vi "VIQA Audit.vi"(6 "Abort":refnum<vi>, 7 "Ignore":T1, 8 "error in (no error)":errorcluster, 9 "AuditSlide":refnum<vi>, 10 "AuditMCLB":refnum<vi>, 11 "My Computer":refnum<vi>) -> (0 "error out":errorcluster, 3 "Audit":T2[](array[typedef]))   [LabVIEW 2018, in "VI Quality.lvlib"]
doc: "This VI audits the project items given the filter criteria"
uses:
  VI Quality.lvlib
  Controls/VIQA Audit.ctl
  Controls/VIQA Audit Ignore.ctl
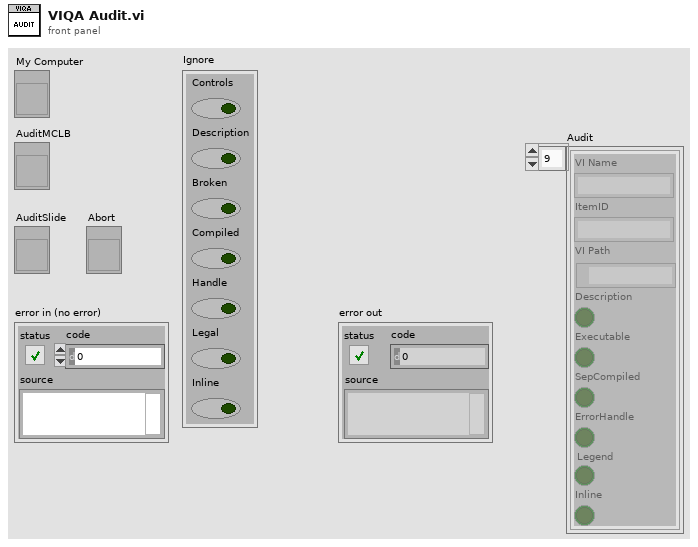
[diagram p1: front panel]
types:
  T1 = typedef "VI Quality.lvlib/VIQA Audit Ignore.ctl" = cluster{"Controls":bool, "Description":bool, "Broken":bool, "Compiled":bool, "Handle":bool, "Legal":bool, "Inline":bool}
  T2 = typedef "VI Quality.lvlib/VIQA Audit.ctl" = cluster{"VI Name":string, "ItemID":string, "VI Path":path, "Description":bool, "Executable":bool, "SepCompiled":bool, "ErrorHandle":bool, "Legend":bool, "Inline":bool}
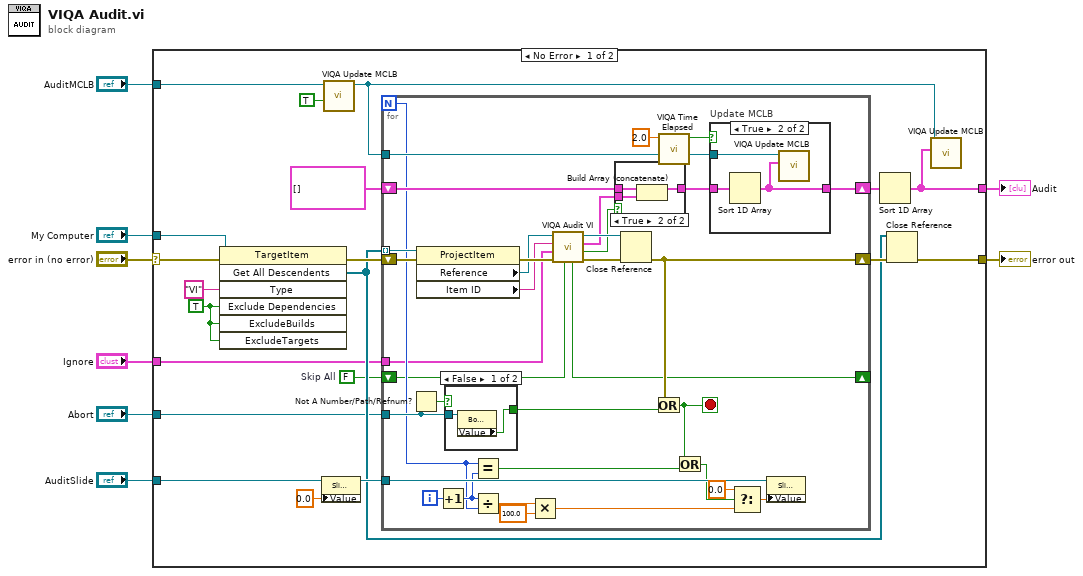
[diagram p0: block diagram]
diagram:
  n1 = case shown="No Error" "error in (no error)" {
    selector: "error in (no error)" -> [w24 w73]
    tunnel: "My Computer" -> [w25 _]
    tunnel: [w12 _] -> w7
    tunnel: [w17 w73] -> w5
    tunnel: "AuditMCLB" -> [w14 _]
    tunnel: "AuditSlide" -> [w23 _]
    tunnel: "Abort" -> [w15 _]
    tunnel: "Ignore" -> [w9 _]
    frame No Error {
      w10 = FALSE  # Skip All
      w27 = TRUE ("ExcludeDependencies")
      n2 = invoke class="TargetItem" method="Get All Descendents"(reference=w25, error in=w24, "Type"="VI", "Exclude Dependencies"=w27, "ExcludeBuilds"=w27, "ExcludeTargets"=w27) -> (error out=w28:errorcluster, "All Descendents"=w16:refnum<vi>[])  [unwired: 1 in, 5 out]
      n3 = property class="Slide (strict)"(reference=w23, "Value"=0.0) -> (reference out=w22:refnum<vi>)  [unwired: 1 in, 1 out]
      n4 = call "VIQA Update MCLB.vi"("Reset TopLeft? (F)"=TRUE, "MCLB"=w14) -> ("dup MCLB"=w11:refnum<vi>)  [unwired: 8 in, 1 out]
      n5 = for {
        N -> [w41]
        tunnel: w16 -> [w61] mode=indexing
        tunnel: w22 -> [w60]
        shift-right: [w44] -> w18
        shift-left: w28 -> [w62]
        shift-right: [w53] -> w19
        shift-left: T2[] [] ("sorted array") -> [w56]
        tunnel: w11 -> [w55]
        tunnel: w15 -> [w47]
        shift-right: [w35] -> _
        shift-left: w10 -> [w36]
        tunnel: w9 -> [w38]
        i -> [w59]
        stop <- w29 stop-if-true
        n6 = Not A Number/Path/Refnum?(number/path/refnum=w47) -> (NaN/Path/Refnum?=w46:bool)
        n7 = property class="ProjectItem"(reference=w61, error in=w62) -> (error out=w39:errorcluster, "Reference"=w37:refnum<vi>, "Item ID"=w34:string)  [unwired: 1 out]
        n8 = Increment(x=w59) -> (x+1=w42:i32)
        n9 = case shown="False" w46 {
          tunnel: w47 -> [w64 _]
          tunnel: [w63 _] -> w45
          frame False {
            n10 = property class="Bool (strict)"(reference=w64) -> ("Value"=w63:bool)  [unwired: 1 in, 2 out]
          }
          frame True {
          }
        }
        n11 = Equal?(x=w41, y=w42) -> (x = y?=w40:bool)
        n12 = Divide(x=w42, y=w41) -> (x/y=w58:dbl)
        n13 = Multiply(x=w58, y=100.0 ("x")) -> (x*y=w48:dbl)
        n14 = call "VIQA Audit VI.vi"("Pwrd Skip All? (F)"=w36, "error in (no error)"=w39, "Ignore"=w38, "Item ID"=w34, "VI Refnum"=w37) -> ("error out"=w33:errorcluster, "Valid?"=w30:bool, "Item"=w31:T2, "dup VI Refnum"=w32:refnum<vi>, "Pwrd Skip All?"=w35:bool)  [unwired: 2 in]
        n15 = case shown="True" w30 {
          tunnel: w56 -> [w69 w72]
          tunnel: w31 -> [_ w71]
          tunnel: [w69 w70] -> w54
          frame False {
          }
          frame True {
            n16 = Build Array (concatenate)(w72, w71) -> (w70:T2[])
          }
        }
        n17 = Close Reference(reference=w32, error in (no error)=w33) -> (error out=w44:errorcluster)
        n18 = Or(x=w44, y=w45) -> (x .or. y?=w29:bool)
        n19 = call "VIQA Time Elapsed.vi"("Duration (1 sec)"=2.0) -> ("Time Has Elapsed?"=w51:bool)  [unwired: 9 in, 1 out]
        n20 = Or(x=w29, y=w40) -> (x .or. y?=w43:bool)
        n21 = case "Update MCLB" shown="True" w51 {
          tunnel: w54 -> [w65 w67]
          tunnel: w55 -> [_ w68]
          tunnel: [w65 w66] -> w53
          frame False {
          }
          frame True {
            n22 = Sort 1D Array(array=w67) -> (sorted array=w66:T2[])
            n23 = call "VIQA Update MCLB.vi"("Items"=w66, "MCLB"=w68) -> ()  [unwired: 8 in, 2 out]
          }
        }
        n24 = Select(t=0.0 ("f"), s=w43, f=w48) -> (s? t:f=w50:dbl)
        n25 = property class="Slide (strict)"(reference=w60, "Value"=w50) -> ()  [unwired: 1 in, 2 out]
      }
      n26 = Sort 1D Array(array=w19) -> (sorted array=w12:T2[])
      n27 = Close Reference(reference=w16, error in (no error)=w18) -> (error out=w17:errorcluster)
      n28 = call "VIQA Update MCLB.vi"("Items"=w12, "MCLB"=w11) -> ()  [unwired: 8 in, 2 out]
    }
    frame Error {
    }
  }
  "Audit" <- w7
  "error out" <- w5
